vi "Sort.vi"(2 "n":i32, 3 "Real":sgl[](array[numeric])=[0.0, 0.0, 0.0, 0.0, 0.0, 0.0, 0.0, 0.0, 0.0, 0.0, 0.0, 0.0, 0.0, 0.0, 0.0, 0.0, 0.0, 0.0, 0.0, 0.0]) -> (1 "Sorted A":sgl[](array[numeric]))   [LabVIEW 2020]
uses:
  <vilib>/rvi/Emulation/niFpgaGetClockAttributes.vi
  <vilib>/rvi/Emulation/niFpgaSctlEmulationGetInTimedLoop.vi
  <vilib>/rvi/Emulation/niFpgaEmulationReportErrorSimple.vi
  <vilib>/rvi/Emulation/niFpgaCriticalErrorInLSC.vi
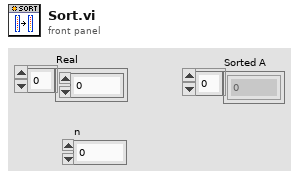
[diagram p1: front panel]
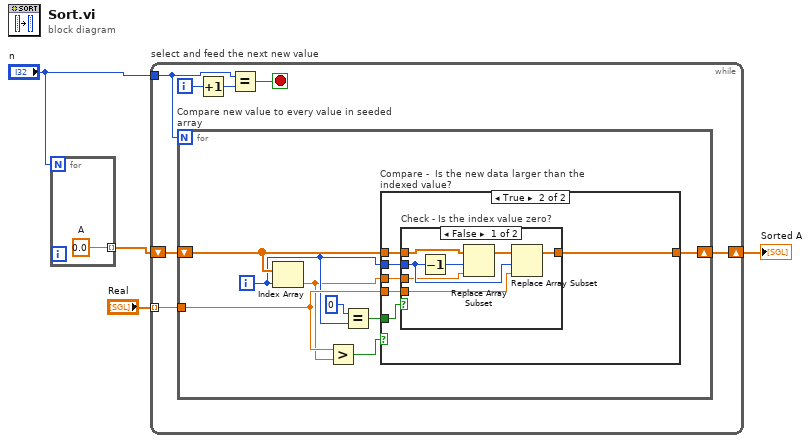
[diagram p0: block diagram]
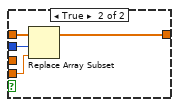
[diagram p3: hidden frame]
diagram:
  n1 = for {
    N: "n" -> [_]
    tunnel: [w5] -> w3 mode=indexing
    w5 = sgl 0.0  # A
  }
  n2 = while "select and feed the next new value" {
    shift-right: [w11] -> w4
    shift-left: w3 -> [w12]
    tunnel: "n" -> [w8]
    tunnel: "Real" -> [w9] mode=indexing
    i -> [w7]
    stop <- w10 stop-if-true
    n3 = for "Compare new value to every value in seeded array" {
      N: w8 -> [_]
      tunnel: w9 -> [w18]
      shift-right: [w17] -> w11
      shift-left: w12 -> [w19]
      i -> [w16]
      n4 = Index Array(array=w19, index=w16) -> (element=w13:sgl)
      n5 = Greater?(x=w18, y=w13) -> (0:w20:bool)
      n6 = Equal?(x=0, y=w16) -> (x = y?=w14:bool)
      n7 = case "Compare -  Is the new data larger than the indexed value?" shown="True" w20 {
        tunnel: w19 -> [w21 w26]
        tunnel: w14 -> [_ w27]
        tunnel: w18 -> [_ w25]
        tunnel: w16 -> [_ w24]
        tunnel: [w21 w23] -> w17
        tunnel: w13 -> [_ w22]
        frame False {
        }
        frame True {
          n8 = case "Check - Is the index value zero?" shown="False" w27 {
            tunnel: w26 -> [w30 w38]
            tunnel: w25 -> [w33 w37]
            tunnel: w24 -> [w29 w35]
            tunnel: [w32 w36] -> w23
            tunnel: w22 -> [w28 _]
            frame False {
              n9 = Decrement(x=w29) -> (x-1=w31:i32)
              n10 = Replace Array Subset(array=w30, new element=w28, index=w31) -> (w34:sgl[])
              n11 = Replace Array Subset(array=w34, new element=w33, index=w29) -> (w32:sgl[])
            }
            frame True {
              n12 = Replace Array Subset(array=w38, new element=w37, index=w35) -> (w36:sgl[])
            }
          }
        }
      }
    }
    n13 = Increment(x=w7) -> (x+1=w6:i32)
    n14 = Equal?(x=w8, y=w6) -> (x = y?=w10:bool)
  }
  "Sorted A" <- w4
